vi "LUCS001RT_GPS_RS232_Readx62.vi"(8 "error in":errorcluster, 9 "FPGA VI Reference In":refnum<k20>) -> (0 "error out":errorcluster, 1 "FPGA VI Reference Out":refnum<k20>, 3 "x62?":bool, 5 "unsigned 8bit integer":u8 format="%02x")   [LabVIEW 2020]
uses:
  <vilib>/rvi/interface/nirviMethod/nirviMethod.xnode
  sbRIO-9612/SourceCodeFPGA/LUCS002FPGA_Main.vi
  SourceCode_Host/SourceCode_Host/FPGA Bitfiles/LUCS002h.lvproj_FPGA Target_LUCS002FPGA_Main.vi.lvbit
  <vilib>/FPGAPlugInAG/sbRIO-9612/niLvFpga_ReadFifo_sbRIO-9612.vi
  <vilib>/rvi/errors/niLvFpgaMergeErrorWithErrorCode.vi
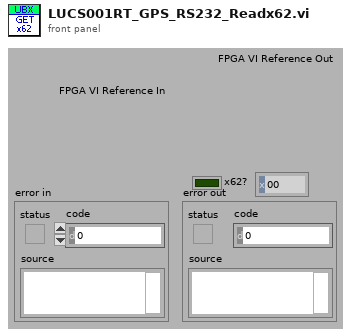
[diagram p1: front panel]
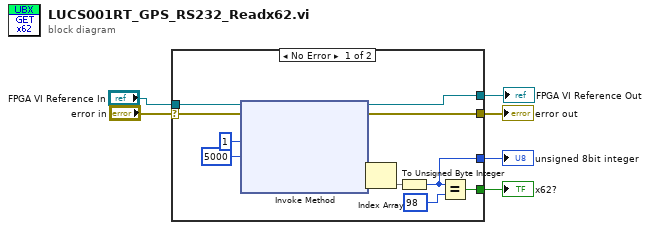
[diagram p0: block diagram]
diagram:
  n1 = case shown="No Error" "error in" {
    selector: "error in" -> [w14 w18]
    tunnel: [w17 _] -> w1
    tunnel: [w16 w18] -> w6
    tunnel: "FPGA VI Reference In" -> [w15 _]
    tunnel: [w8 _] -> w4
    tunnel: [w7 _] -> w3
    frame No Error {
      n2 = xnode "Invoke Method"("FPGA VI Reference In"=w15, "error in"=w14, "Number of Elements"=u32 1, "Timeout (ms)"=5000) -> ("FPGA VI Reference Out"=w17:refnum<k20>, "error out"=w16:errorcluster, "Data"=w11:void[])  [unwired: 1 out]
      n3 = Index Array(array=w11) -> (element=w10)  [unwired: 1 in]
      n4 = To Unsigned Byte Integer(number=w10) -> (unsigned 8bit integer=w7:u8)
      n5 = Equal?(x=w7, y=u8 98 ("element")) -> (x = y?=w8:bool)
    }
    frame Error {
    }
  }
  "x62?" <- w4
  "error out" <- w6
  "unsigned 8bit integer" <- w3
  "FPGA VI Reference Out" <- w1
